vi "ImportedVideoConversion.vi"() -> ()   [LabVIEW 2019]
uses:
  RGB_To_Gray DLL Project/Project RGBToGray VI/RGBToGray.dll
  GrayToRGBAlternative DLL Project/VI Project/GrayToRGBAlternative.dll
panel:
  out "Frame Data":T1
  out "Elapsed time for RGB to Gray in sec":dbl
  out "RGB Frame":T2(plugin-control)
  out "Gray Frame":T2(plugin-control)
  out "Elapsed time for Gray to RGB in sec":dbl
  out "Original Frame":T2(plugin-control)
  in  "Available Colormaps":T3
  in  "Stop":bool
  out "Progress Bar":i32(slide) max=677 scale=-1.0..677.0
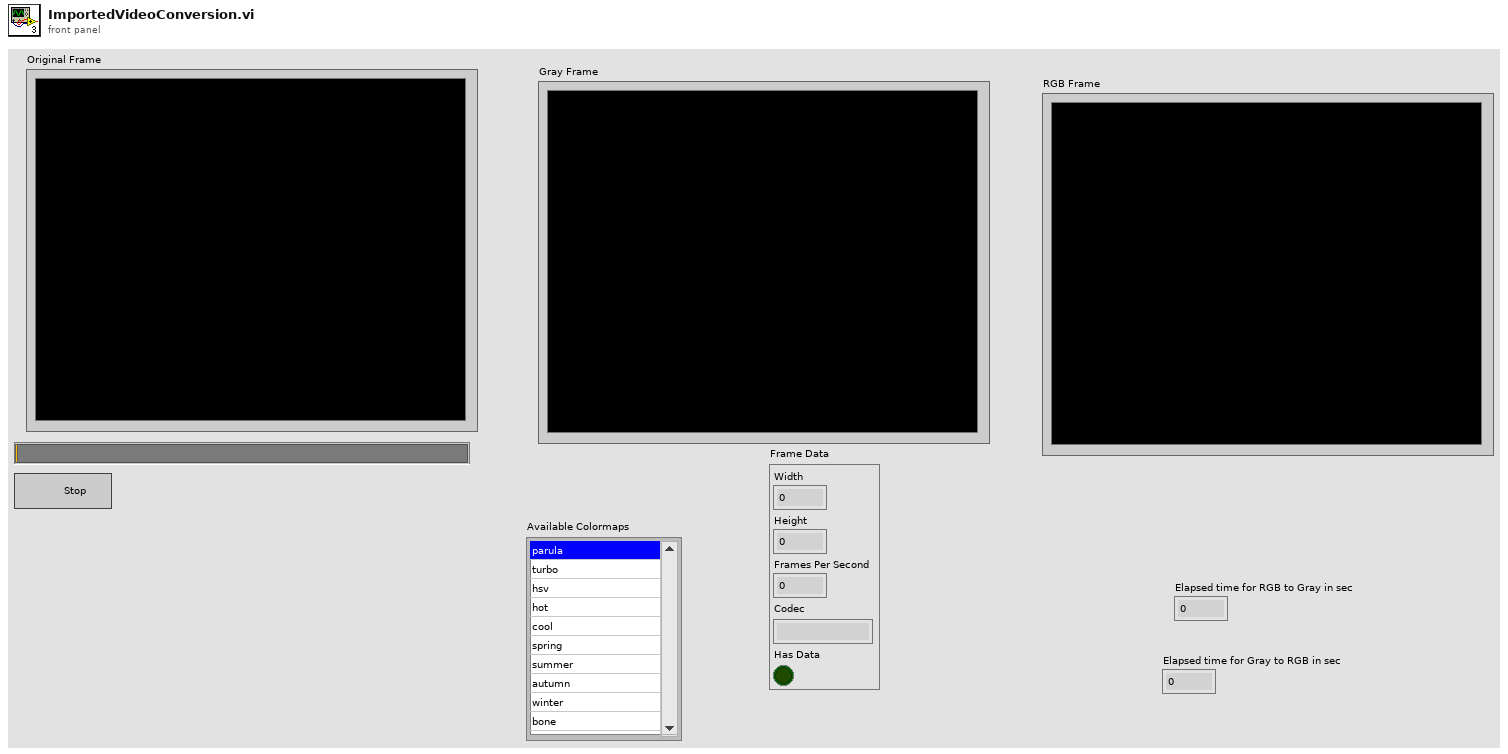
[diagram p1: front panel]
types:
  T1 = cluster{"Width":u32, "Height":u32, "Frames Per Second":u32, "Codec":string, "Has Data":bool}
  T2 = typedef "IMAQ Image.ctl" = refnum<image>
  T3 = typedef "Control 1.ctl" = i32
  T4 = typedef "Image Type" = u32
  T5 = typedef "IMAQ AVI2 Refnum.ctl" = refnum<k20>
  T6 = enum32{"Map Pixel Pointer", "Unmap Pixel Pointer", "Get Pixels Infos"}
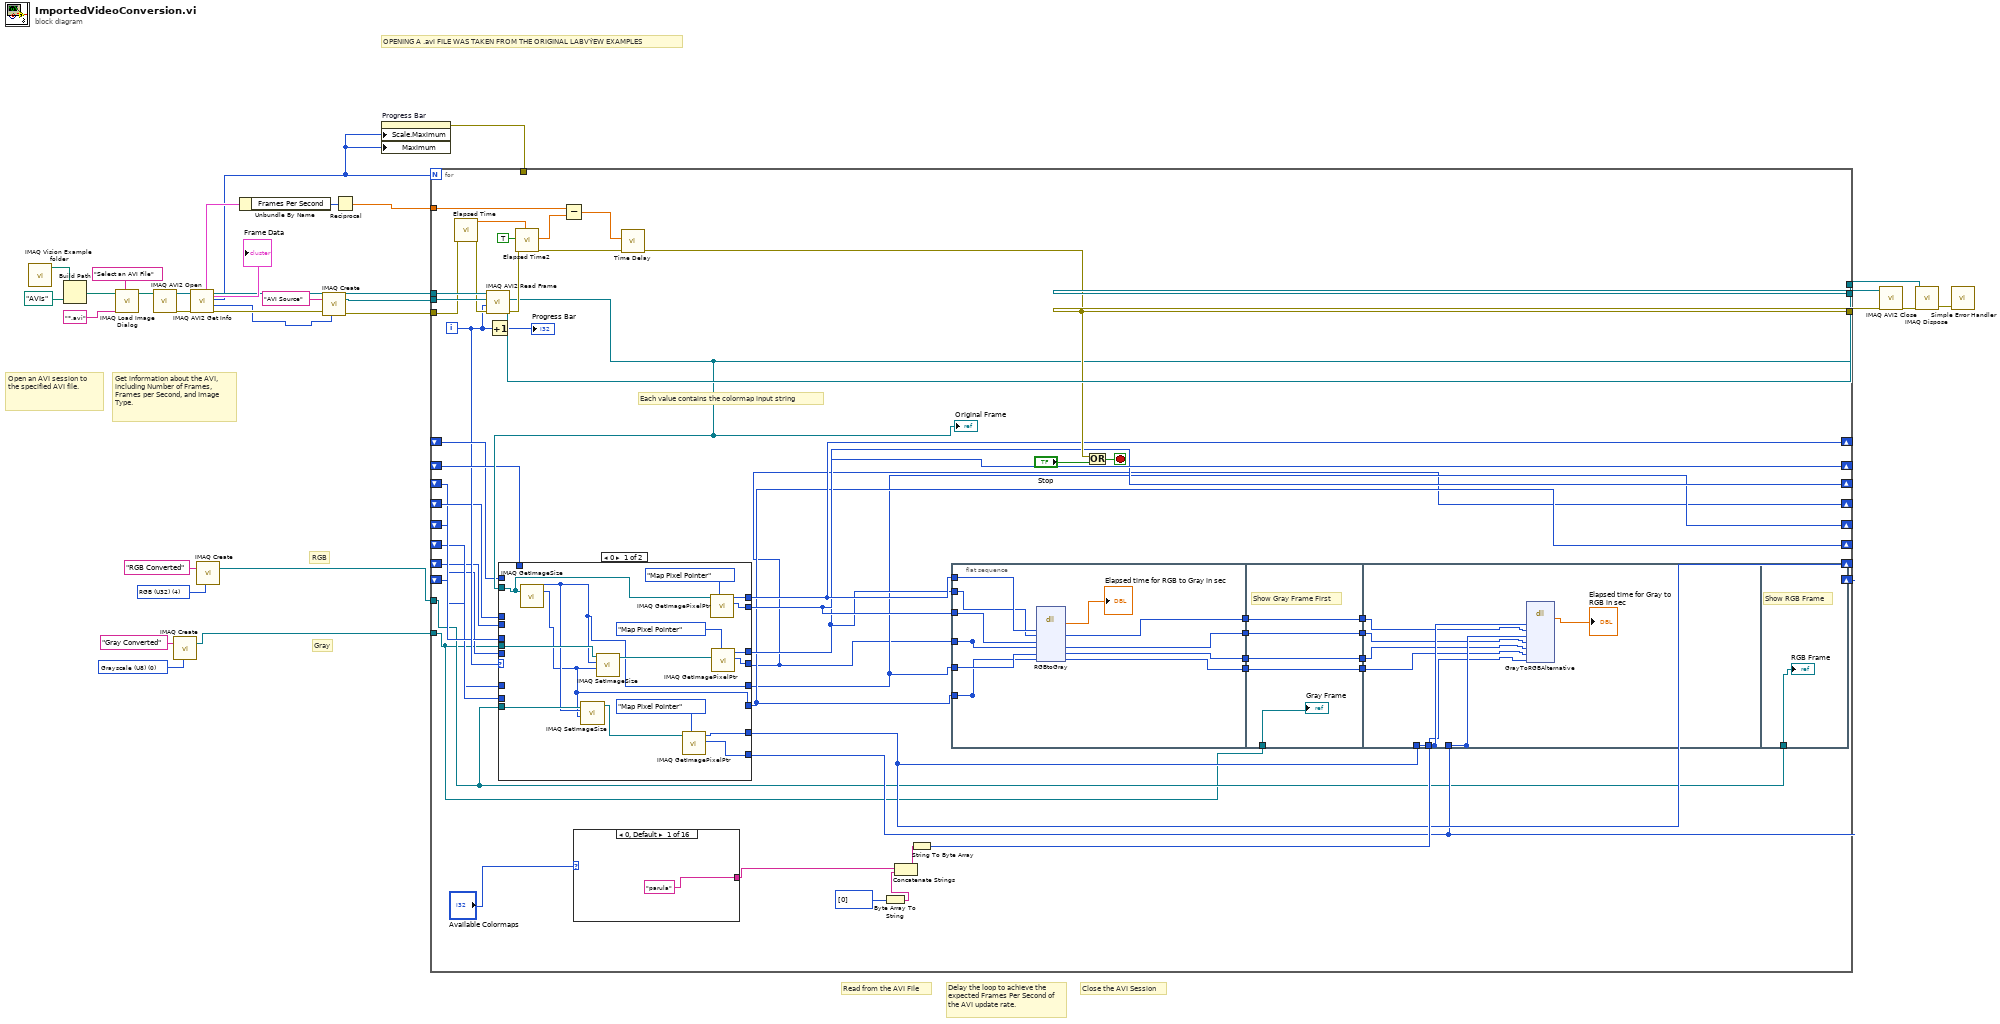
[diagram p0: block diagram]
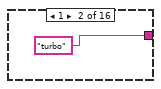
[diagram p3: hidden frame]
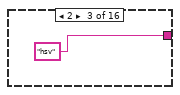
[diagram p4: hidden frame]
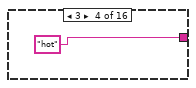
[diagram p5: hidden frame]
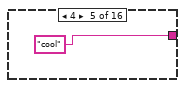
[diagram p6: hidden frame]
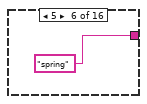
[diagram p7: hidden frame]
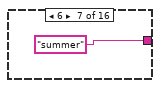
[diagram p8: hidden frame]
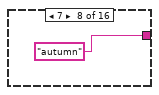
[diagram p9: hidden frame]
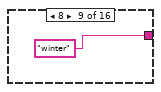
[diagram p10: hidden frame]
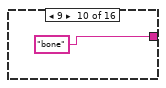
[diagram p11: hidden frame]
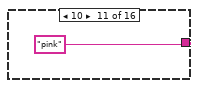
[diagram p12: hidden frame]
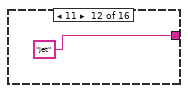
[diagram p13: hidden frame]
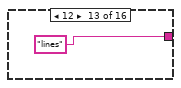
[diagram p14: hidden frame]
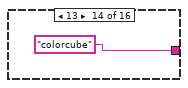
[diagram p15: hidden frame]
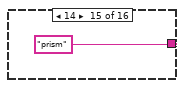
[diagram p16: hidden frame]
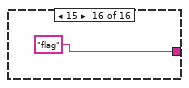
[diagram p17: hidden frame]
diagram:
  w2 = T4 0 items=["Grayscale (U8)", "Grayscale (I16)", "Grayscale (SGL)", "Complex (CSG)", "RGB (U32)", "HSL (U32)", "RGB (U64)", "Grayscale (U16)"] ("Image Type")
  w4 = T4 4 items=["Grayscale (U8)", "Grayscale (I16)", "Grayscale (SGL)", "Complex (CSG)", "RGB (U32)", "HSL (U32)", "RGB (U64)", "Grayscale (U16)"] ("Image Type")
  # "Gray"
  # "RGB"
  # "OPENING A .avi FILE WAS TAKEN FROM THE ORIGINAL LABVÝEW EXAMPLES"
  # "Close the AVI Session"
  # "Read from the AVI File"
  # "Get information about the AVI, including Number of Frames, Frames per Second, and Image Type."
  # "Open an AVI session to the specified AVI file."
  # "Delay the loop to achieve the expected Frames Per Second of the AVI update rate."
  n1 = call "IMAQ Vision Example folder.vi"() -> ("Example Image Path"=w15:path)  [unwired: 11 in]
  n2 = Build Path(base path=w15, name or relative path=path "AVIs") -> (appended path=w12:path)
  n3 = call "IMAQ Load Image Dialog"("Prompt"="Select an AVI File" ("prompt"), "Pattern"="*.avi", "Start Path"=w12) -> ("Path"=w11:path)  [unwired: 6 in, 2 out]
  n4 = call "IMAQ AVI2 Open"("AVI File Path"=w11) -> ("error out"=w27:errorcluster, "AVI Refnum"=w26:T5)  [unwired: 2 in, 7 out]
  n5 = call "IMAQ Create"("Image Name"="Gray Converted", "Image Type"=w2) -> ("New Image"=w1:T2)  [unwired: 3 in, 1 out]
  n6 = call "IMAQ AVI2 Get Info"("error in (no error)"=w27, "AVI Refnum"=w26) -> ("error out"=w23:errorcluster, "Image Type"=w7:T4, "Number of Frames"=w9:u32, "AVI Refnum (duplicate)"=w20:T5, "Frame Data"=w28:T1)  [unwired: 5 out]
  "Frame Data" <- w28
  n7 = call "IMAQ Create"("Image Name"="RGB Converted", "Image Type"=w4) -> ("New Image"=w5:T2)  [unwired: 3 in, 1 out]
  n8 = Unbundle By Name(w28) -> ("Frames Per Second"=w17:u32)
  n9 = call "IMAQ Create"("Image Name"="AVI Source", "Image Type"=w7, "error in (no error)"=w23) -> ("New Image"=w21:T2, "error out"=w22:errorcluster)  [unwired: 1 in, 1 out]
  n10 = Reciprocal(x=w17) -> (1/x=w16:dbl)
  n11 = property on="Progress Bar" class="Slide (strict)"("Scale.Maximum"=w9, "Maximum"=w9) -> (error out=w8:errorcluster)  [unwired: 2 in, 1 out]
  n12 = for {
    N: w9 -> [_]
    tunnel: w21 -> [w79]
    tunnel: [w78] -> w24
    tunnel: [w68] -> w25
    tunnel: w22 -> [w77]
    tunnel: w20 -> [w80]
    tunnel: [w59] -> w18
    tunnel: w16 -> [w75]
    tunnel: w8 -> [_]
    tunnel: w5 -> [w34]
    tunnel: w1 -> [w33]
    shift-right: [w40] -> _
    shift-left: _ -> [w57]
    shift-right: [w39] -> _
    shift-left: _ -> [w58]
    shift-right: [w38] -> _
    shift-left: _ -> [w54]
    shift-right: [w35] -> _
    shift-left: _ -> [w55]
    shift-right: [w36] -> _
    shift-left: _ -> [w52]
    shift-right: [w37] -> _
    shift-left: _ -> [w53]
    shift-right: [w42] -> _
    shift-left: _ -> [w50]
    shift-right: [w41] -> _
    shift-left: _ -> [w51]
    i -> [w56]
    stop <- w66 stop-if-true
    # "Each value contains the colormap input string"
    n13 = call "Elapsed Time"("error in (no error)"=w77) -> ("Present (s)"=w73:dbl, "error out"=w76:errorcluster)  [unwired: 11 in, 6 out]
    n14 = call "IMAQ AVI2 Read Frame"("error in (no error)"=w76, "Frame Number"=w56, "Image"=w79, "AVI Refnum"=w80) -> ("error out"=w71:errorcluster, "Image Out"=w59:T2, "AVI Refnum (duplicate)"=w78:T5)  [unwired: 5 out]
    "Original Frame" <- w59
    n15 = Increment(x=w56) -> (x+1=→"Progress Bar":i32)
    n16 = case shown="0" w56 {
      tunnel: w59 -> [w110 _]
      tunnel: w33 -> [w116 _]
      tunnel: w34 -> [w115 _]
      tunnel: [w114 w123] -> w42
      tunnel: [w113 w122] -> w41
      tunnel: [w112 w127] -> w38
      tunnel: [w111 w126] -> w35
      tunnel: [w109 w125] -> w36
      tunnel: [w108 w124] -> w37
      tunnel: [w107 w129] -> w40
      tunnel: [w106 w128] -> w39
      tunnel: w57 -> [_ w129]
      tunnel: w58 -> [_ w128]
      tunnel: w54 -> [_ w127]
      tunnel: w55 -> [_ w126]
      tunnel: w52 -> [_ w125]
      tunnel: w53 -> [_ w124]
      tunnel: w50 -> [_ w123]
      tunnel: w51 -> [_ w122]
      frame 0 {
        n17 = call "IMAQ GetImageSize"("Image"=w110) -> ("Y Resolution"=w108:i32, "X Resolution"=w109:i32)  [unwired: 3 in, 1 out]
        n18 = call "IMAQ SetImageSize"("Y Resolution"=w108, "X Resolution"=w109, "Image"=w115) -> ("Image Out"=w119:T2)  [unwired: 2 in, 1 out]
        n19 = call "IMAQ SetImageSize"("Y Resolution"=w108, "X Resolution"=w109, "Image"=w116) -> ("Image Out"=w117:T2)  [unwired: 2 in, 1 out]
        n20 = call "IMAQ GetImagePixelPtr"("Function"=T6."Map Pixel Pointer", "Image"=w119) -> ("LineWidth(Pixels)"=w113:i32, "Pixel Pointer out"=w114:u64)  [unwired: 4 in, 4 out]
        n21 = call "IMAQ GetImagePixelPtr"("Function"=T6."Map Pixel Pointer", "Image"=w110) -> ("LineWidth(Pixels)"=w106:i32, "Pixel Pointer out"=w107:u64)  [unwired: 4 in, 4 out]
        n22 = call "IMAQ GetImagePixelPtr"("Function"=T6."Map Pixel Pointer", "Image"=w117) -> ("LineWidth(Pixels)"=w111:i32, "Pixel Pointer out"=w112:u64)  [unwired: 4 in, 4 out]
      }
      frame 1, Default {
      }
    }
    n23 = call "Elapsed Time2"("Reset"=TRUE, "error in (no error)"=w71, "Set Start Time (s)"=w73) -> ("Elapsed Time (s)"=w70:dbl, "error out"=w69:errorcluster)  [unwired: 9 in, 6 out]
    n24 = Subtract(x=w75, y=w70) -> (x-y=w74:dbl)
    n25 = case shown="0, Default" "Available Colormaps" {
      tunnel: ["parula" "turbo" "hsv" "hot" "cool" "spring" "summer" "autumn" "winter" "bone" "pink" "jet" "lines" "colorcube" "prism" "flag"] -> w60
      frame 0, Default {
      }
      frame 1 {
      }
      frame 2 {
      }
      frame 3 {
      }
      frame 4 {
      }
      frame 5 {
      }
      frame 6 {
      }
      frame 7 {
      }
      frame 8 {
      }
      frame 9 {
      }
      frame 10 {
      }
      frame 11 {
      }
      frame 12 {
      }
      frame 13 {
      }
      frame 14 {
      }
      frame 15 {
      }
    }
    n26 = call "Time Delay"("error in (no error)"=w69, "Delay Time (s)"=w74) -> ("error out"=w68:errorcluster)  [unwired: 9 in]
    n27 = Byte Array To String(unsigned byte array=u8[] [0]) -> (string=w62:string)
    n28 = Concatenate Strings(w60, w62) -> (w61:string)
    n29 = String To Byte Array(string=w61) -> (unsigned byte array=w43:u8[])
    n30 = flat-sequence {
      tunnel: [w84] -> w49
      tunnel: [w83] -> w48
      tunnel: w40 -> [w91]
      tunnel: w38 -> [w90]
      tunnel: w39 -> [w89]
      tunnel: w35 -> [w88]
      tunnel: w36 -> [w87]
      tunnel: [w86] -> _
      tunnel: [w88] -> _
      tunnel: w37 -> [w86]
      tunnel: [w82] -> w32
      tunnel: [w81] -> w31
      tunnel: w49 -> [w96]
      tunnel: [w96] -> w47
      tunnel: w48 -> [w95]
      tunnel: [w95] -> w46
      tunnel: [w94] -> w45
      tunnel: [w93] -> w44
      tunnel: w33 -> [w92]
      tunnel: w32 -> [w94]
      tunnel: w31 -> [w93]
      tunnel: w43 -> [w98]
      tunnel: w47 -> [w103]
      tunnel: w46 -> [w101]
      tunnel: w45 -> [w100]
      tunnel: w44 -> [w99]
      tunnel: [w104] -> _
      tunnel: [w102] -> _
      tunnel: w42 -> [w104]
      tunnel: w41 -> [w102]
      tunnel: w34 -> [w105]
      frame #0 {
        n31 = dll-call lib="C:/Users/byald/Desktop/EE-433 Project Group1/RGB_To_Gray DLL Project/Project RGBToGray VI/RGBToGray.dll" fn="RGBtoGray"("RGBImage"=w91, "GrayImage"=w90, "LVLineWidthRGB"=w89, "LVLineWidthGray"=w88, "LVWidth"=w87, "LVHeight"=w86) -> ("return type"=→"Elapsed time for RGB to Gray in sec":dbl, "GrayImage"=w84:u64, "LVLineWidthGray"=w83:i32, "LVWidth"=w82:i32, "LVHeight"=w81:i32)  [unwired: 5 in, 2 out]
      }
      frame #1 {
        # "Show Gray Frame First"
        "Gray Frame" <- w92
      }
      frame #2 {
        n32 = dll-call lib="C:/Users/byald/Desktop/EE-433 Project Group1/GrayToRGBAlternative DLL Project/VI Project/GrayToRGBAlternative.dll" fn="GrayToRGBAlternative"("RGBImage"=w104, "GrayImage"=w103, "LVLineWidthRGB"=w102, "LVLineWidthGray"=w101, "LVWidth"=w100, "LVHeight"=w99, "ColorMap"=w98) -> ("return type"=→"Elapsed time for Gray to RGB in sec":dbl)  [unwired: 10 in, 2 out]
      }
      frame #3 {
        # "Show RGB Frame"
        "RGB Frame" <- w105
      }
    }
    n33 = Or(x=w68, y="Stop") -> (x .or. y?=w66:bool)
  }
  n34 = call "IMAQ AVI2 Close"("error in (no error)"=w25, "AVI Refnum"=w24) -> ("error out"=w19:errorcluster)  [unwired: 9 out]
  n35 = call "IMAQ Dispose"("Image"=w18, "error in (no error)"=w19) -> ("error out"=w29:errorcluster)  [unwired: 1 in, 3 out]
  n36 = call <vilib>:"Simple Error Handler.vi"("error in (no error)"=w29) -> ()  [unwired: 1 in, 8 out]
